vi "Get Temp Feedback--Method.vi"(8 "error in (no error)":errorcluster, 10 "Temp Units":T1, 11 "Simulated Thermal Process Controller in":refnum<class "Simulated Thermal Process Controller.lvclass">) -> (0 "error out":errorcluster, 2 "Temp Feedback":dbl, 3 "Simulated Thermal Process Controller out":refnum<class "Simulated Thermal Process Controller.lvclass">)   [LabVIEW 2024, in "Simulated Thermal Process Controller.lvclass"]
uses:
  Simulated Thermal Process Controller.lvclass
  Process Controller/Controls/Temperature Units--Enum.ctl
  Simulated Thermal Process Controller.lvclass/Simulated Thermal Process Controller.ctl
  Process Controller/_Thermal Process Controller.lvclass
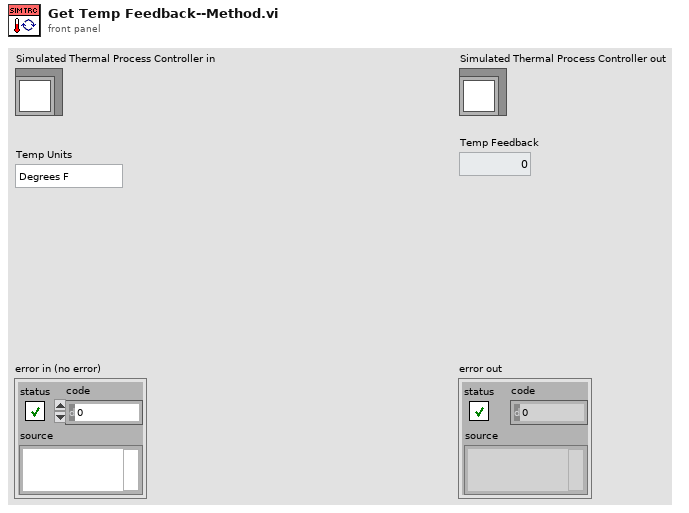
[diagram p1: front panel]
types:
  T1 = typedef "_Thermal Process Controller.lvclass/Temperature Units--Enum.ctl" = enum16{"Degrees F", "Degrees C", "Degrees K"}
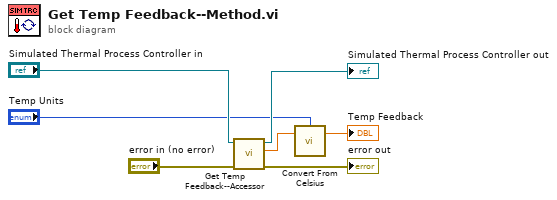
[diagram p0: block diagram]
diagram:
  n1 = call "Get Temp Feedback--Accessor.vi"("error in (no error)"="error in (no error)", "Simulated Thermal Process Controller in"="Simulated Thermal Process Controller in") -> ("error out"=→"error out":errorcluster, "Temp Feedback"=w3:dbl, "Simulated Thermal Process Controller out"=→"Simulated Thermal Process Controller out":refnum<class "Simulated Thermal Process Controller.lvclass">)  [unwired: 7 in]
  n2 = call "Convert From Celsius.vi"("Temp In"=w3, "Temp Units"="Temp Units") -> ("Temp Out"=→"Temp Feedback":dbl)  [unwired: 3 in]
